vi "Read OpenFPWhenCreated Key.vi"(8 "Error In":errorcluster) -> (0 "Error Out":errorcluster, 3 "Open Front Panel When Created?":enum32{"Yes", "No"}(ring))   [LabVIEW 2022 SP3]
doc: "This VI reads the value of the \"OpenFrontPanelWhenNewViCreated\" Windows Registry Key.\n\nThe key (the setting) is found at Computer\\HKEY_CURRENT_USER\\Software\\NewViFromTemplate_LabVIEW_IDE_Extension.\n\nIf the key doesn't exist, this VI creates it, as well as the \"OpenFrontPanelWhenNewViCreated\" value.\n\nIf the key exists, but the \"OpenFrontPanelWhenNewViCreated\" value doesn't, this VI creates the value and assigns it the default value of \"Yes\"."
uses:
  <vilib>/registry/registry.llb/Write Registry Value Simple STR.vi
  <vilib>/registry/registry.llb/Read Registry Value Simple STR.vi
panel:
  # "Development\nControls or indicators that are useful for development or testing, but which are not outputs of the VI."
  # "Input\nInputs to the VI"
  # "Output\nOutputs of the VI"
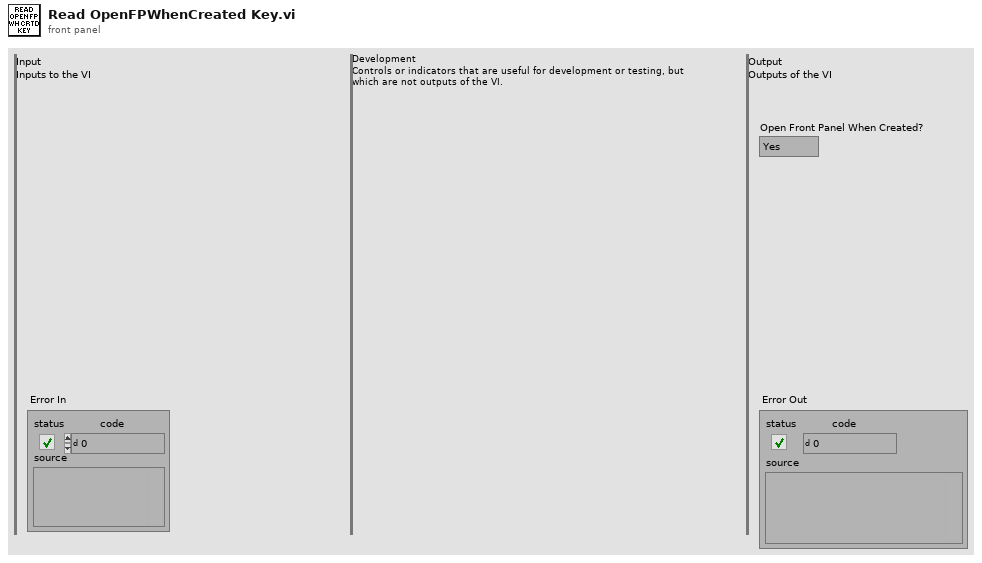
[diagram p1: front panel]
types:
  T1 = typedef "Registry RtKey.ctl" = enum32{"HKEY_CLASSES_ROOT", "HKEY_CURRENT_USER", "HKEY_LOCAL_MACHINE", "HKEY_USERS", "HKEY_PERFORMANCE_DATA", "HKEY_CURRENT_CONFIG", "HKEY_DYN_DATA"}
  T2 = typedef "Registry refnum.ctl" = refnum<k1>
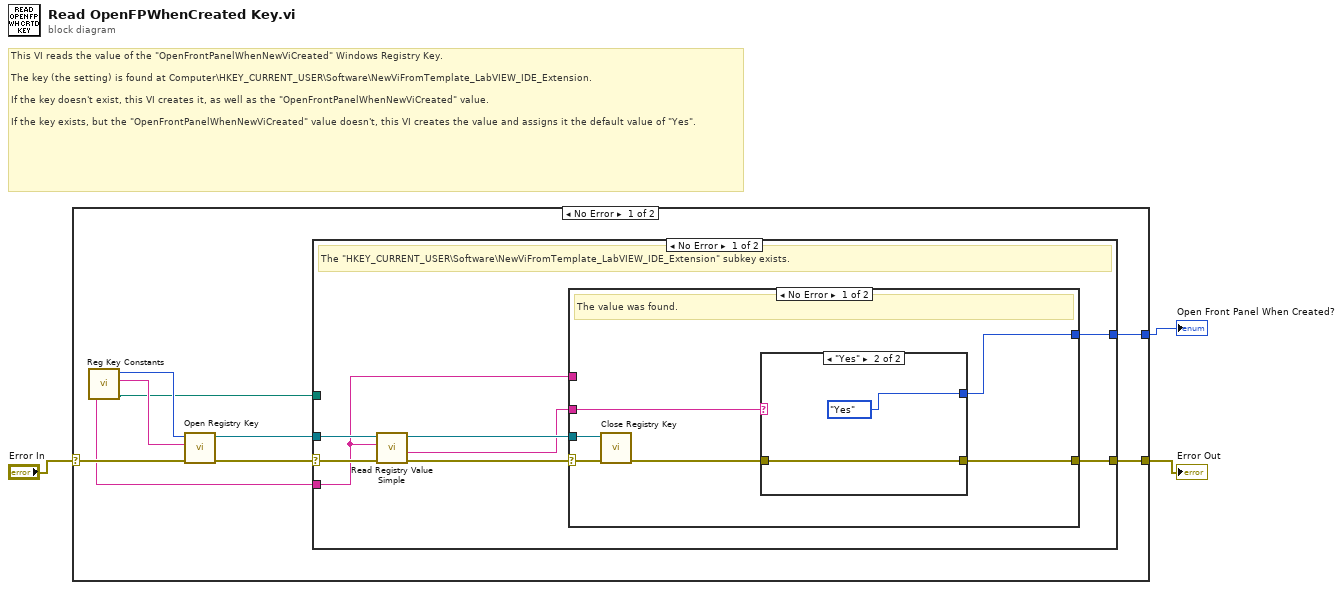
[diagram p0: block diagram]
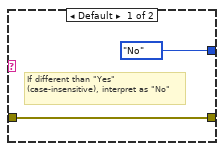
[diagram p2: hidden frame]
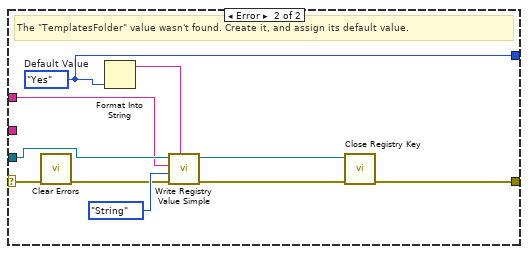
[diagram p3: hidden frame]
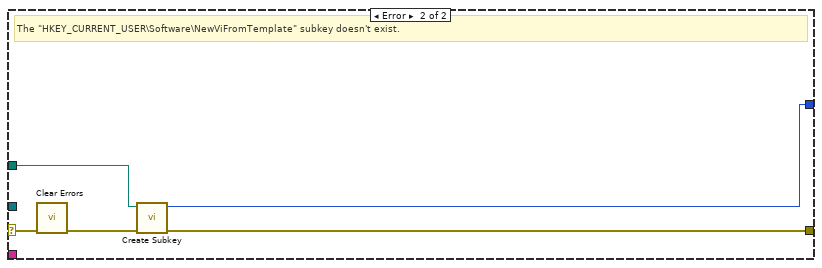
[diagram p4: hidden frame]
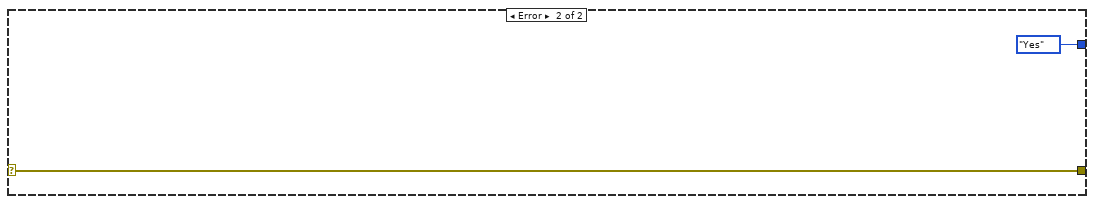
[diagram p5: hidden frame]
diagram:
  # "This VI reads the value of the \"OpenFrontPanelWhenNewViCreated\" Windows Registry Key.\n\nThe key (the setting) is found at Computer\\HKEY_CURRENT_USER\\Software\\NewViFromTemplate_LabVIEW_IDE_Extension.\n\nIf the key doesn't exist, this VI creates it, as well as the \"OpenFrontPanelWhenNewViCreated\" value.\n\nIf the key exists, but the \"OpenFrontPanelWhenNewViCreated\" value doesn't, this VI creates the value and assigns it the default value of \"Yes\"."
  n1 = case shown="No Error" "Error In" {
    selector: "Error In" -> [w12 w47]
    tunnel: [w10 w47] -> w2
    tunnel: [w4 enum32{"Yes", "No"}."Yes" ("The default value of the \"Open FP When Created?\" setting")] -> w1
    frame No Error {
      n2 = call "Reg Key Constants.vi"() -> ("Default Templates Folder"=w6:path, "Subkey Path"=w7:string, "Root Key"=w8:T1, "Name of OpenFrontPanelWhenNewViCreated Value"=w5:string)  [unwired: 3 in, 1 out]
      n3 = call <vilib>:"Open Registry Key.vi"("error in (no error)"=w12, "subkey"=w7, "root key (HKEY_LOCAL_MACHINE)"=w8) -> ("error out"=w11:errorcluster, "refnum out"=w9:T2)  [unwired: 7 in]
      n4 = case shown="No Error" w11 {
        selector: w11 -> [w20 w45]
        tunnel: [w18 w44] -> w10
        tunnel: w9 -> [w16 _]
        tunnel: w5 -> [w14 _]
        tunnel: w6 -> [_ w43]
        tunnel: [w13 w41] -> w4
        frame No Error {
          # "The \"HKEY_CURRENT_USER\\Software\\NewViFromTemplate_LabVIEW_IDE_Extension\" subkey exists."
          n5 = call-poly <vilib>:"Read Registry Value Simple.vi"("error in (no error)"=w20, "value"=w14, "refnum"=w16) -> ("error out"=w19:errorcluster, "String/Binary data"=w15:string, "refnum out"=w17:T2)  [unwired: 3 in, 1 out]
          n6 = case shown="No Error" w19 {
            selector: w19 -> [w26 w39]
            tunnel: [w23 w35] -> w18
            tunnel: w17 -> [w24 w38]
            tunnel: w15 -> [w22 _]
            tunnel: w14 -> [_ w33]
            tunnel: [w21 w31] -> w13
            frame No Error {
              # "The value was found."
              n7 = call <vilib>:"Close Registry Key.vi"("error in (no error)"=w26, "refnum"=w24) -> ("error out"=w25:errorcluster)  [unwired: 5 in]
              n8 = case shown="\"Yes\"" w22 {
                tunnel: w25 -> [w28 w30]
                tunnel: [w28 w30] -> w23
                tunnel: [enum32{"Yes", "No"}."No" ("Default Value") enum32{"Yes", "No"}."Yes" ("Default Value")] -> w21
                frame Default {
                  # "If different than \"Yes\" (case-insensitive), interpret as \"No\""
                }
                frame "Yes" {
                }
              }
            }
            frame Error {
              w31 = enum32{"Yes", "No"}."Yes"  # Default Value
              # "The \"TemplatesFolder\" value wasn't found. Create it, and assign its default value."
              n9 = call <vilib>:"Clear Errors.vi"("error in (no error)"=w39) -> ("error out"=w37:errorcluster)  [unwired: 5 in, 1 out]
              n10 = Format Into String(w31) -> (resulting string=w32:string)  [unwired: 3 in, 1 out]
              n11 = call-poly <vilib>:"Write Registry Value Simple.vi"("String/Binary data"=w32, "error in (no error)"=w37, "simple data type"=enum16{"String", "Binary", "DWORD"}."String", "value"=w33, "refnum"=w38) -> ("error out"=w36:errorcluster, "refnum out"=w34:T2)  [unwired: 3 in]
              n12 = call <vilib>:"Close Registry Key.vi"("error in (no error)"=w36, "refnum"=w34) -> ("error out"=w35:errorcluster)  [unwired: 5 in]
            }
          }
        }
        frame Error {
          # "The \"HKEY_CURRENT_USER\\Software\\NewViFromTemplate\" subkey doesn't exist."
          n13 = call <vilib>:"Clear Errors.vi"("error in (no error)"=w45) -> ("error out"=w42:errorcluster)  [unwired: 5 in, 1 out]
          n14 = call "Create Subkey.vi"("Error In"=w42, "Default Templates Folder Path"=w43) -> ("Error Out"=w44:errorcluster, "The default value of the \"Open FP When Created?\" setting"=w41:enum32{"Yes", "No"})  [unwired: 8 in]
        }
      }
    }
    frame Error {
    }
  }
  "Error Out" <- w2
  "Open Front Panel When Created?" <- w1
